vi "Read DBPath.vi"(8 "error in (no error)":errorcluster, 11 "Messages Actor in":refnum<class "Messages Actor.lvclass">) -> (0 "error out":errorcluster, 2 "DBPath":path, 3 "Messages Actor out":refnum<class "Messages Actor.lvclass">)   [LabVIEW 2020, in "Messages Actor.lvlib" / "Messages Actor.lvclass"]
uses:
  Messages Actor.lvclass
  Messages Actor.lvclass/Messages Actor.ctl
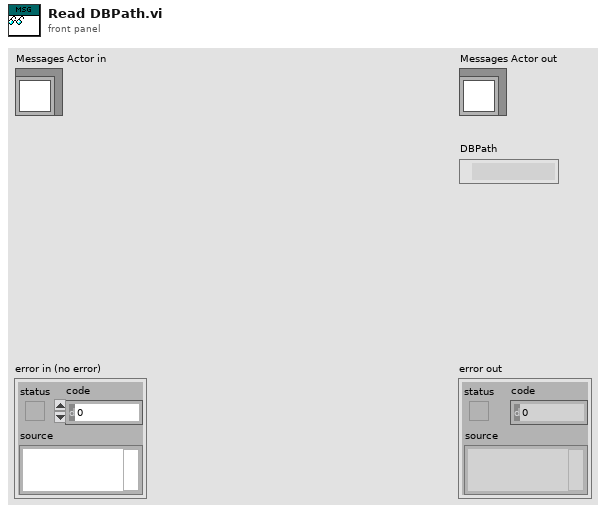
[diagram p1: front panel]
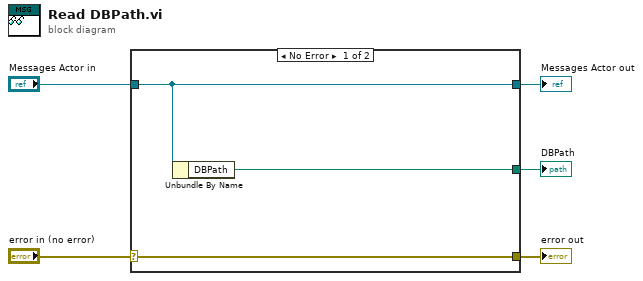
[diagram p0: block diagram]
diagram:
  n1 = case shown="No Error" "error in (no error)" {
    selector: "error in (no error)" -> [w8 w9]
    tunnel: [w8 w9] -> w4
    tunnel: [w7 w10] -> w2
    tunnel: "Messages Actor in" -> [w7 w10]
    tunnel: [w6 _] -> w1
    frame No Error {
      n2 = Unbundle By Name(w7) -> ("DBPath"=w6:path)
    }
    frame Error {
    }
  }
  "error out" <- w4
  "Messages Actor out" <- w2
  "DBPath" <- w1
